vi "TagDashboard.vi"(7 "Name(\"\" to use uuid)":string="UI.Dashboard") -> ()   [LabVIEW 2020, in "CSM-TagDashboard.lvlib"]
doc: "------------- lvcsm -------------\n[CSMStates]\nItem 0 = \"Idle\"\nItem 1 = \"CSM Documentation\"\nItem 2 = \"VI Reference\"\nItem 3 = \"Error Handler\"\nItem 4 = \"Critical Error\"\nItem 5 = \"Target Timeout Error\"\nItem 6 = \"Target Error\"\nItem 7 = \"Async Response\"\nItem 8 = \"Response\"\nItem 9 = \"Async Message Posted\"\nItem 10 = \"Initialize Core Data\"\nItem 11 = \"Exit\"\nItem 12 = \"Data: Initialize\"\nItem 13 = \"Data: Update Indicators\"\nItem 14 = \"Data: Load Attributes\"\nItem 15 = \"Data: Save Attributes\"\nItem 16 = \"Data: Cleanup\"\nItem 17 = \"Macro: Initialize\"\nItem 18 = \"Macro: Exit\"\nItem 19 = \"API: Start Refreshing\"\nItem 20 = \"API: Stop Refreshing\"\nItem 21 = \"Action: Insert TestStandOI\"\nItem 22 = \"Action: Relocate Boolean Switchs\"\nItem 23 = \"Action: 修改bool状态\"\nItem 24 = \"Action: Sync Bool Value with DB\"\nItem 25 = \"Action: 更新当前测试名称\"\nItem 26 = \"Action: Refresh Waveform\"\nItem 27 = \"Action: Refresh Check\"\nItem 28 = \"Action: Resize Array\"\n\n[CSMStatus]\nItem 0 = \"Error Occurred@Error Handler\"\nItem 1 = \"电磁阀状态修改@Action: 修改bool状态\""
uses:
  CSM-TagDashboard.lvlib
  a029ab59-1b26-456a-9f2f-fd23f89c2af1.vi
  67aca029-dc61-4838-a765-978c85277e00.vi
  07294343-d0f4-4418-a8a6-c52ea02f7694.vi
  <userlib>/_NEVSTOP/TagDB/_Support/DataAccess/TagDB Ref to DVR.vi
  <userlib>/_NEVSTOP/Communicable State Machine(CSM)/AdvanceAPI/CSM - Revert Arguments-Safe String.vi
  <userlib>/_NEVSTOP/Communicable State Machine(CSM)/_Shared/Trim Single-line Text.vi
  <userlib>/_NEVSTOP/Communicable State Machine(CSM)/AdvanceAPI/CSM - Make String Arguments Safe.vi
  <userlib>/_NEVSTOP/Communicable State Machine(CSM)/AdvanceAPI/CSM - Break Down Multiple States String.vi
  <userlib>/_NEVSTOP/Communicable State Machine(CSM)/AdvanceAPI/CSM - Compact Multiple States.vi
  <userlib>/_NEVSTOP/Communicable State Machine(CSM)/AdvanceAPI/CSM - Keywords.vi
  <userlib>/_NEVSTOP/Communicable State Machine(CSM)/addons/API-String-Arugments-Support/_Support/Convert API String Arguments to Data(variant).vi
  <userlib>/_NEVSTOP/Communicable State Machine(CSM)/AdvanceAPI/CSM - List Modules.vi
  <userlib>/_NEVSTOP/Communicable State Machine(CSM)/Communicable State Machine.lvlib
  <userlib>/_NEVSTOP/TagDB/TagDB.lvlib
panel:
  out "Tags":string[](array[string])
  out "TagDB":refnum<k1>
  out "Prompt":string="Power by CSM, NEVSTOP-LAB\nUnlicensed Version - 0.0min Trial Left"
  out "Dashboard":T1(array[cluster])
  in  "Num Rows":i16=10
  in  "Num Col":i16=8
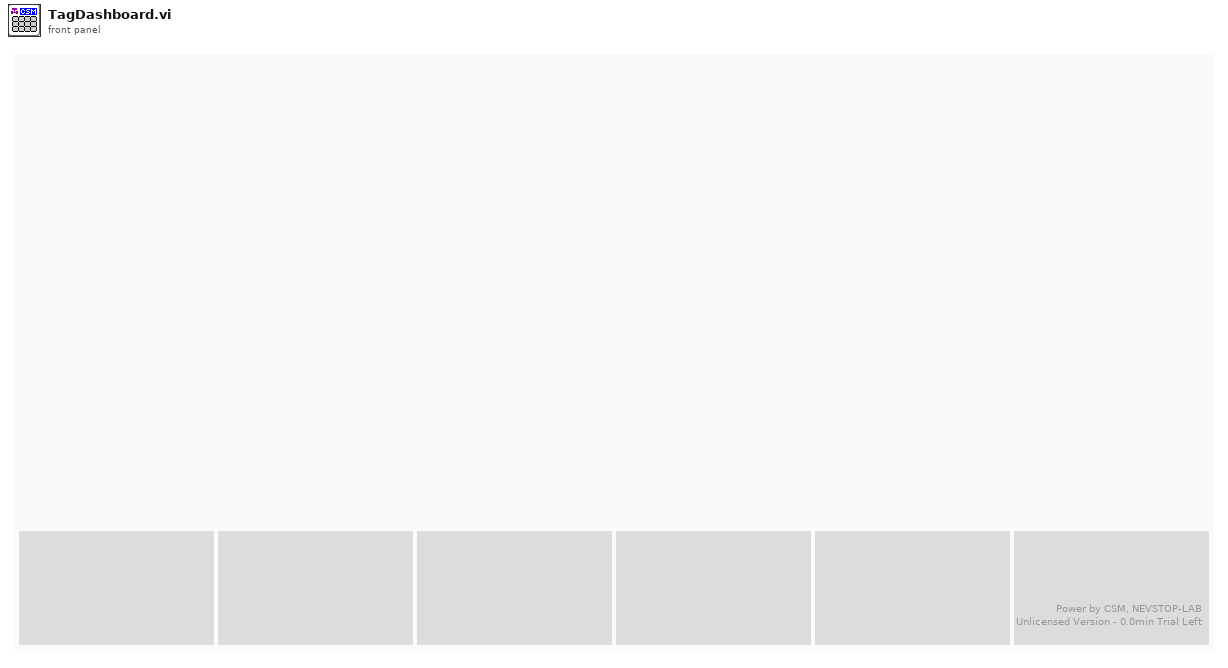
[diagram p1: front panel]
types:
  T1 = cluster{"Label":string, "Value":string, "String":string}[][]
  T2 = cluster{"Label Font Size":i32, "Data Font Size":i32, "String Font Size":i32}
  T3 = cluster{"DataName(dup)":string, "Output String":string, "Unit":string}[][]
  T4 = typedef "LVPositionTypeDef.ctl" = cluster{"Left":i32, "Top":i32}
  T5 = typedef "LVBoundsTypeDef.ctl" = cluster{"Width":u32, "Height":u32}
  T6 = cluster{"Position":T4, "Bounds":T5, "Num Col":i16, "Num Rows":i16, "Cluster":cluster{"Label Font Size":i32, "Data Font Size":i32, "String Font Size":i32}, "Width":u32, "Height":u32}
  T7 = enum32{"Invalid", "Standard", "Closed", "Hidden", "Minimized", "Maximized"}
  T8 = enum32{"invalid app kind", "Development System", "Run Time System", "Student Edition", "Embedded LabVIEW", "Evaluation", "Custom"}
  T9 = typedef "Communicable State Machine.lvlib/_CSM_Response Source Message.ctl" = cluster{"‘State":string, "’Arguments":string, "’Error":errorcluster}
  T10 = cluster{"Current VI Reference":refnum<vi>, "Close Panel on Exit?":bool}
  T11 = cluster{"Core":cluster{"Current VI Reference":refnum<vi>, "Close Panel on Exit?":bool}, "Tags":string[], "Size":cluster{"Cols":i16, "Rows":i16}}
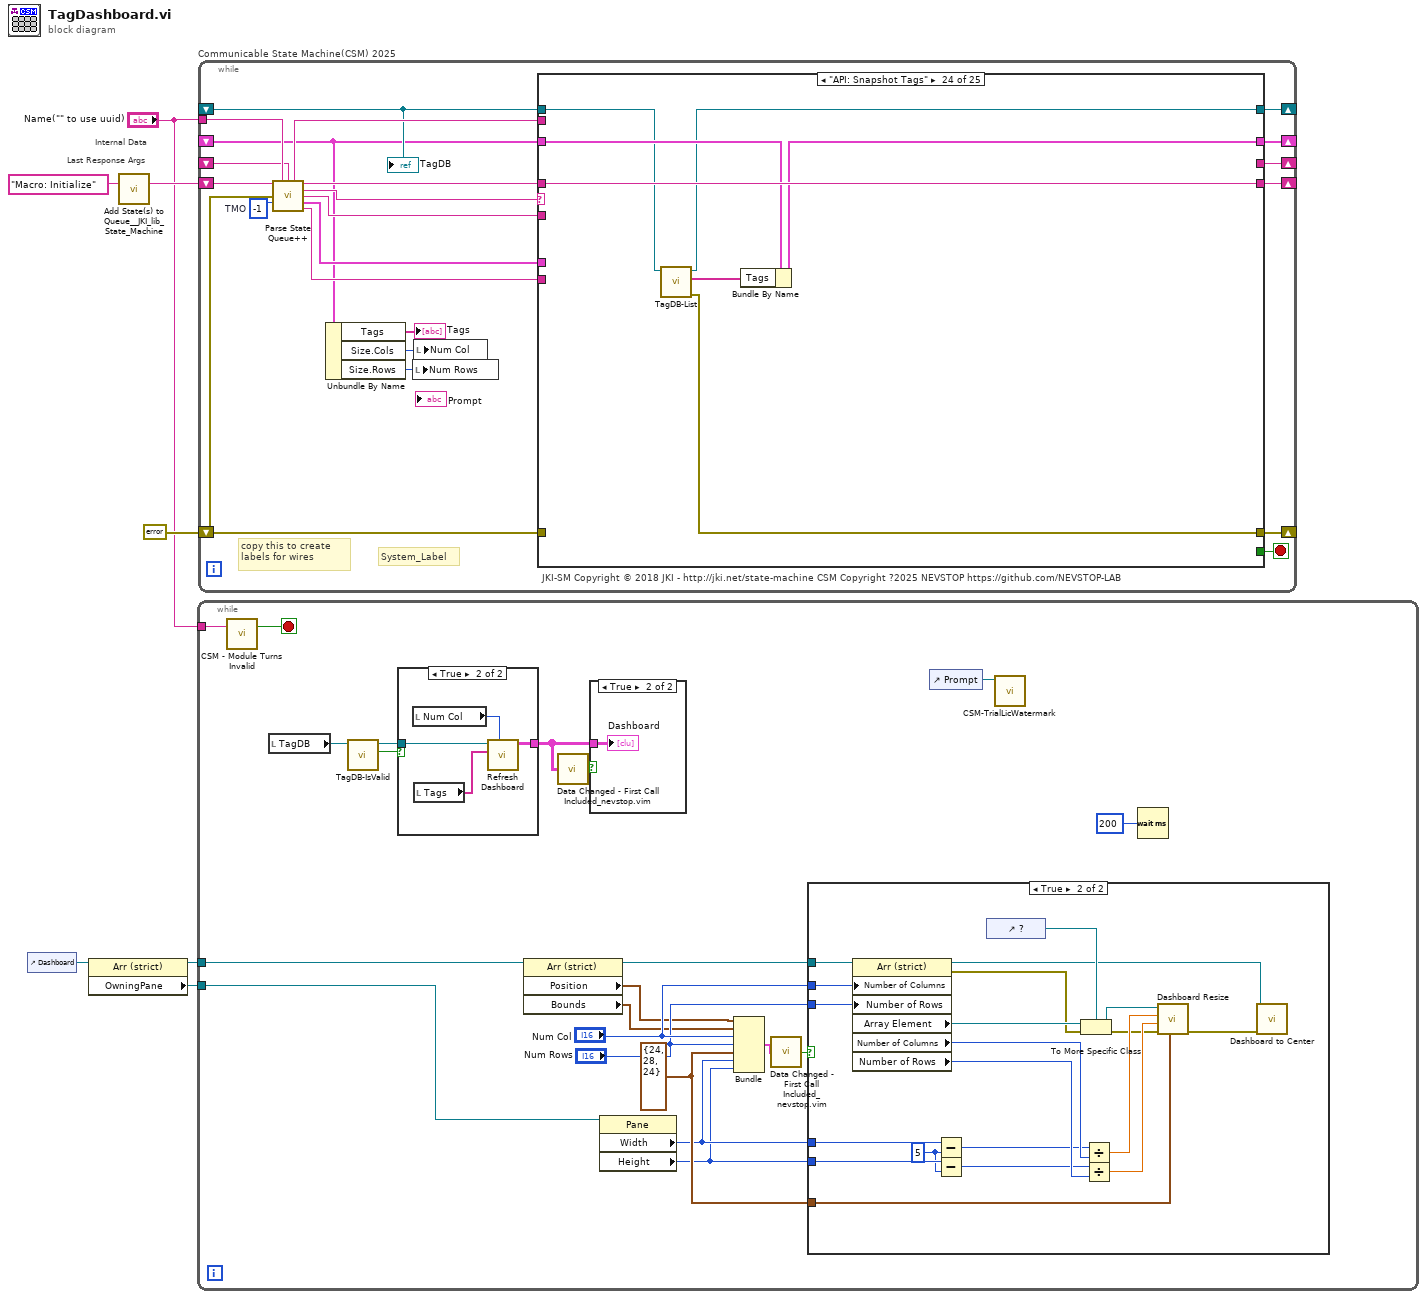
[diagram p0: block diagram]
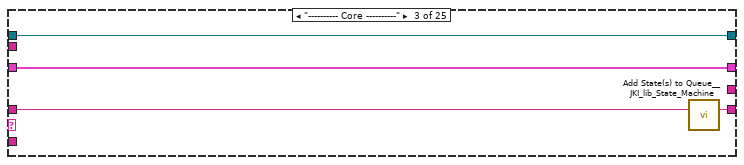
[diagram p7: hidden frame]
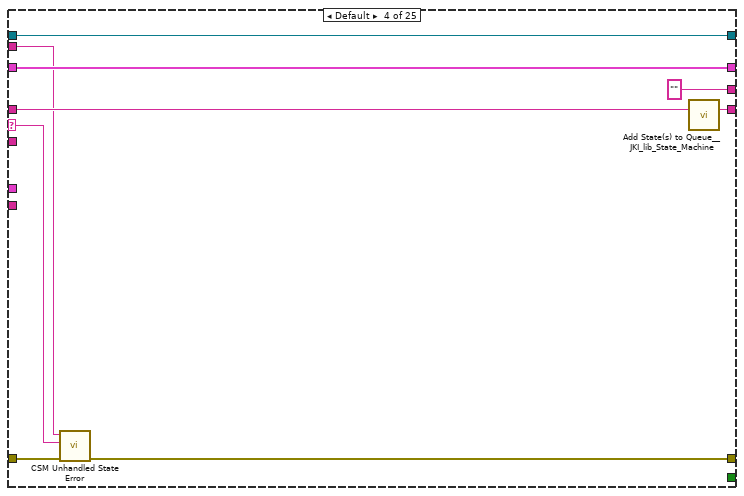
[diagram p8: hidden frame]
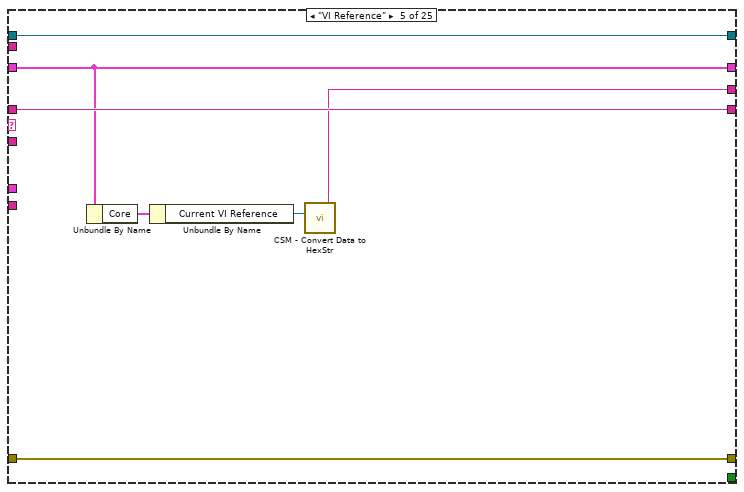
[diagram p9: hidden frame]
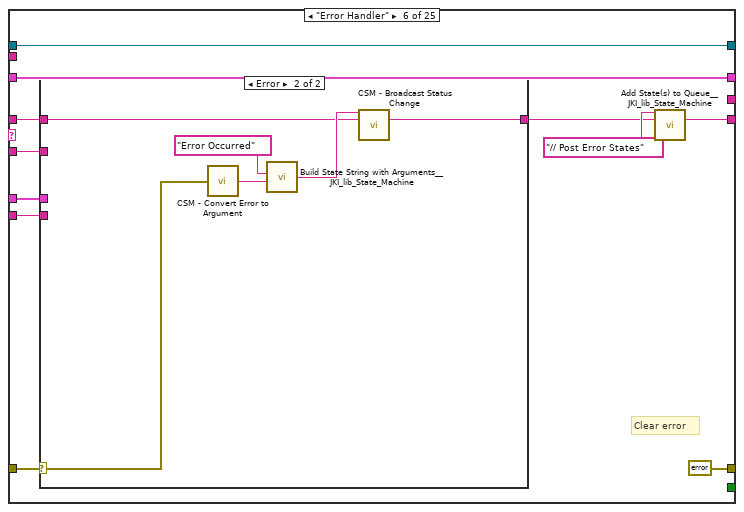
[diagram p10: hidden frame]
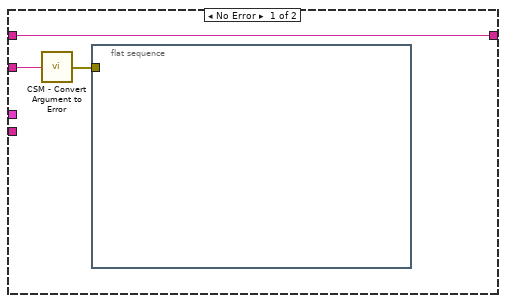
[diagram p11: hidden frame]
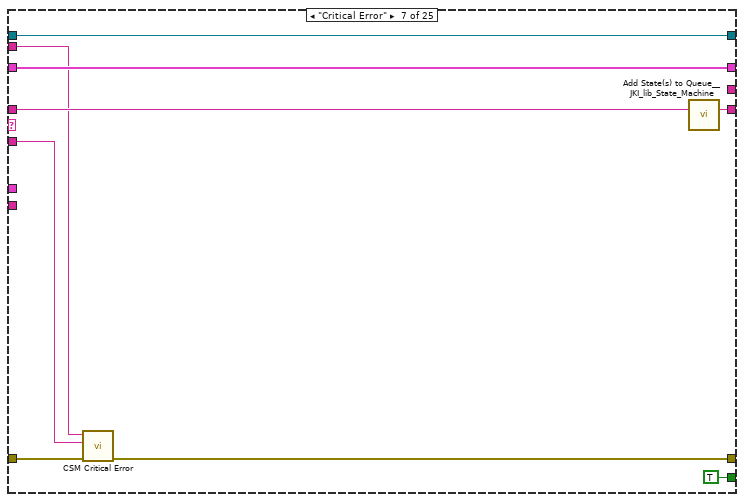
[diagram p12: hidden frame]
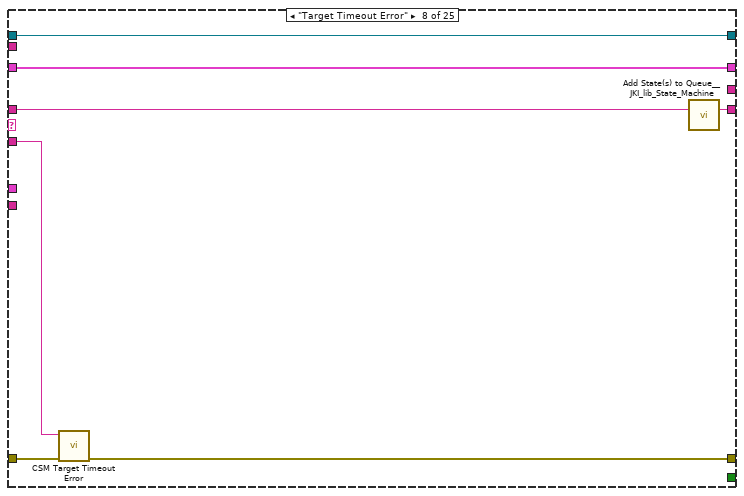
[diagram p13: hidden frame]
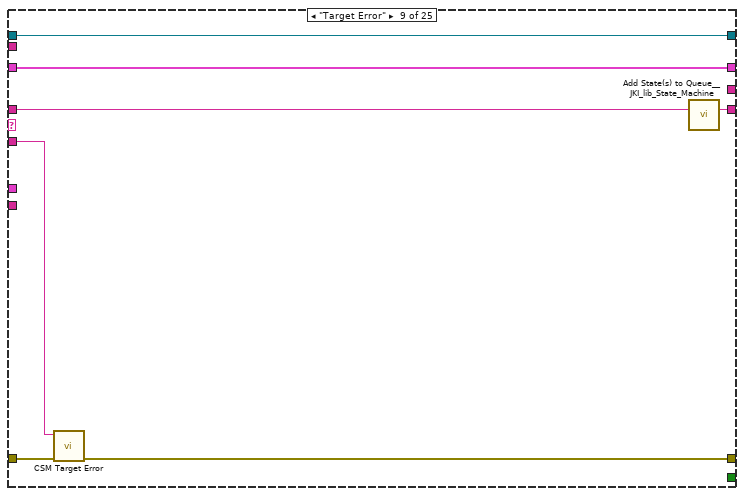
[diagram p14: hidden frame]
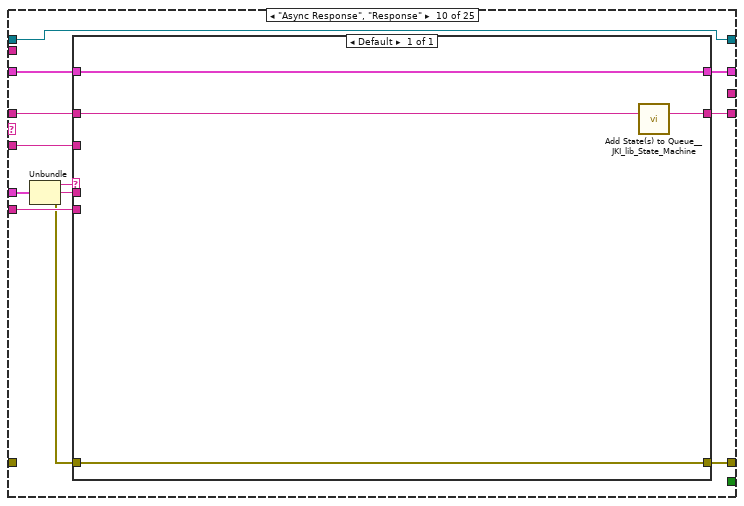
[diagram p15: hidden frame]
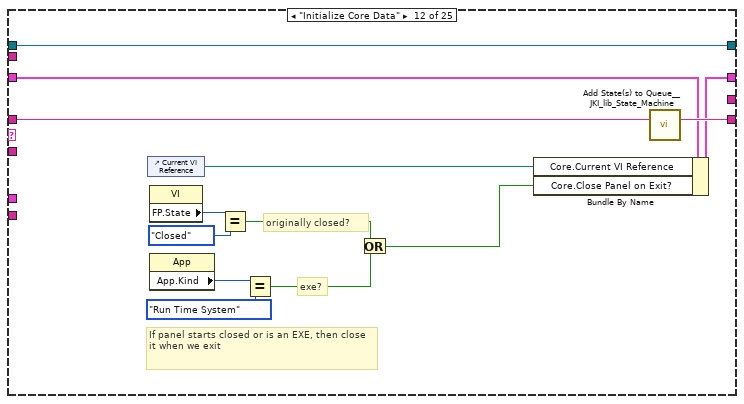
[diagram p17: hidden frame]
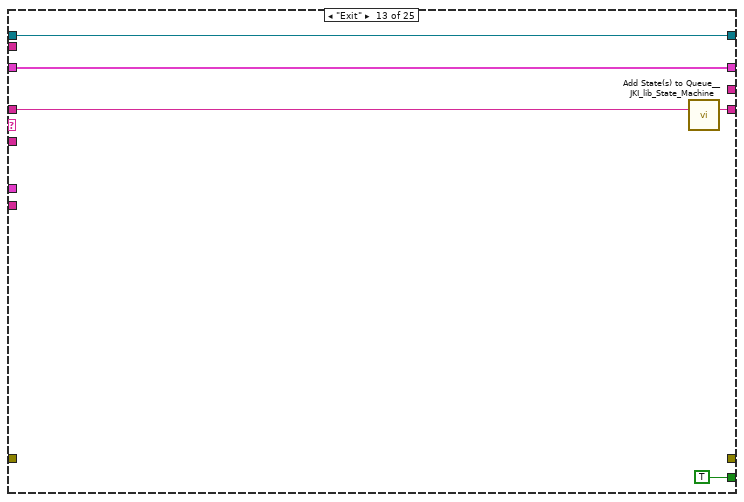
[diagram p18: hidden frame]
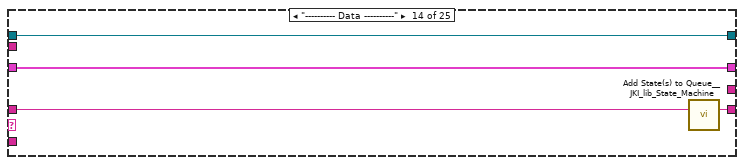
[diagram p19: hidden frame]
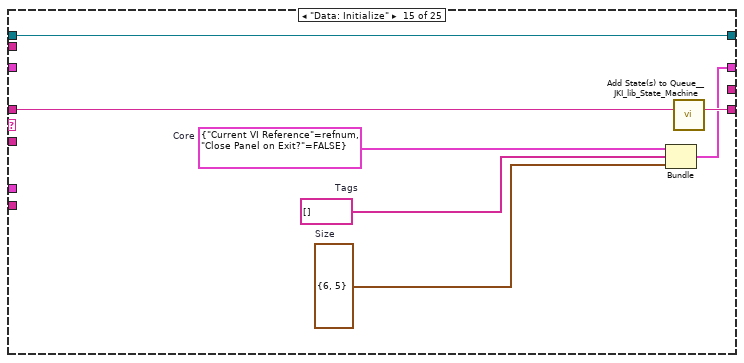
[diagram p20: hidden frame]
diagram:
  # "Last Response Args"
  # "Internal Data"
  n1 = control-ref of="Dashboard"() -> (w4:refnum<vi>)
  n2 = property class="Arr (strict)"(reference=w4) -> (reference out=w3:refnum<vi>, "OwningPane"=w2:refnum<vi>)  [unwired: 1 in, 1 out]
  n3 = call <vilib>:"Add State(s) to Queue__JKI_lib_State_Machine.vi"("State(s) in (\"\")"="Macro: Initialize" ("Init State(\"Macro: Initialize\")")) -> ("States Out"=w7:string)  [unwired: 14 in]
  n4 = while {
    tunnel: "Name(\"\" to use uuid)" -> [w28]
    tunnel: w3 -> [w14]
    tunnel: w2 -> [w13]
    stop <- w27 stop-if-true
    w20 = T2 {"Label Font Size"=24, "Data Font Size"=28, "String Font Size"=24} ("Cluster")
    n5 = call <userlib>:"CSM - Module Turns Invalid.vi"("CSM Name"=w28) -> ("Turn Invalid (Exit)?"=w27:bool)  [unwired: 2 in]
    n6 = local read "TagDB"() -> (w25:refnum<k1>)
    n7 = call <userlib>:"TagDB-IsValid.vi"("TagDB"=w25) -> ("valid TagDB?"=w23:bool, "TagDB(dup)"=w24:refnum<k1>)  [unwired: 8 in, 1 out]
    n8 = case shown="True" w23 {
      tunnel: [_ w33] -> w19
      tunnel: w24 -> [_ w31]
      frame False {
      }
      frame True {
        n9 = local read "Num Col"() -> (w32:i16)
        n10 = local read "Tags"() -> (w30:string[])
        n11 = call "Refresh Dashboard.vi"("Num Col"=w32, "appended array"=w30, "Refnum in"=w31) -> ("Array"=w33:T3)  [unwired: 8 in]
      }
    }
    n12 = property class="Arr (strict)"(reference=w14) -> (reference out=w11:refnum<vi>, "Position"=w9:T4, "Bounds"=w10:T5)  [unwired: 1 in, 1 out]
    n13 = call "Data Changed - First Call Included_nevstop.vim"("Variant"=w19) -> ("Changed"=w18:bool)
    n14 = case shown="True" w18 {
      tunnel: w19 -> [_ w29]
      frame False {
      }
      frame True {
        "Dashboard" <- w29
      }
    }
    n15 = property on="Property Node" class="Pane"(reference=w13) -> ("Width"=w17:u32, "Height"=w16:u32)  [unwired: 1 in, 2 out]
    n16 = Bundle("Position"=w9, "Bounds"=w10, "Num Col"="Num Col", "Num Rows"="Num Rows", "Cluster"=w20, "Width"=w17, "Height"=w16) -> (w15:T6)  [unwired: 1 in]
    n17 = call "Data Changed - First Call Included_nevstop.vim"("Variant"=w15) -> ("Changed"=w8:bool)
    n18 = case shown="True" w8 {
      tunnel: "Num Col" -> [_ w42]
      tunnel: "Num Rows" -> [_ w41]
      tunnel: w20 -> [_ w40]
      tunnel: w11 -> [_ w39]
      tunnel: w17 -> [_ w38]
      tunnel: w16 -> [_ w37]
      frame False {
      }
      frame True {
        w34 = u32 5 ("y")
        n19 = property on="Property Node" class="Arr (strict)"(reference=w39, "Number of Columns"=w42, "Number of Rows"=w41) -> (reference out=w43:refnum<vi>, error out=w51:errorcluster, "Array Element"=w53:refnum<vi>, "Number of Columns"=w52:u32, "Number of Rows"=w50:u32)  [unwired: 1 in]
        n20 = Subtract(x=w38, y=w34) -> (x-y=w36:u32)
        n21 = Subtract(x=w37, y=w34) -> (x-y=w35:u32)
        n22 = control-ref of="?"() -> (w45:refnum<vi>)
        n23 = To More Specific Class(target class=w45, reference=w53, error in=w51) -> (specific class reference=w49:refnum<vi>, error out=w46:errorcluster)
        n24 = Divide(x=w36, y=w52) -> (x/y=w48:dbl)
        n25 = Divide(x=w35, y=w50) -> (x/y=w47:dbl)
        n26 = call "Dashboard Resize.vi"("Cluster"=w40, "error in (no error)"=w46, "Cluster Size:Height"=w47, "Cluster Size:Width"=w48, "ClusterRef"=w49) -> ("error out"=w44:errorcluster)  [unwired: 4 in, 2 out]
        n27 = call "Dashboard to Center.vi"("error in (no error)"=w44, "Control Ref"=w43) -> ()  [unwired: 9 in, 1 out]
      }
    }
    n28 = control-ref of="Prompt"() -> (w12:refnum<vi>)
    n29 = call <userlib>:"CSM-TrialLicWatermark.vi"("TrialLicWatermark"=w12) -> ()  [unwired: 8 in, 3 out]
    n30 = Wait (ms)(milliseconds to wait=u32 200) -> ()  [unwired: 1 out]
  }
  n31 = while "Communicable State Machine(CSM) 2025" {
    shift-right: [w70] -> _
    shift-left: _ -> [w57]
    shift-right: [w73] -> _
    shift-left: errorcluster {"status"=FALSE, "code"=0, "source"=""} ("error out") -> [w60]
    shift-right: [w72] -> _
    shift-left: w7 -> [w74]
    tunnel: "Name(\"\" to use uuid)" -> [w67]
    shift-right: [w68] -> _
    shift-left: _ -> [w62]
    shift-right: [w59] -> _
    shift-left: _ -> [w58]
    stop <- w71 stop-if-true
    w69 = -1  # TMO
    # "JKI-SM Copyright © 2018 JKI - http://jki.net/state-machine CSM Copyright ?2025 NEVSTOP https://github.com/NEVSTOP-LAB"
    # "copy this to create labels for wires"
    # "System_Label"
    n32 = call <userlib>:"Parse State Queue++.vi"("State Queue"=w74, "Name (\"\" to Use UUID)"=w67, "Response Arguments"=w62, "Previous Error"=w60, "Dequeue (1 ms)"=w69) -> ("Name Used"=w61:string, "Remaining States"=w75:string, "Current State"=w63:string, "Arguments"=w64:string, "Additional Information"=w65:T9, "Source CSM"=w66:string)  [unwired: 5 in]
    n33 = Unbundle By Name(w57) -> ("Tags"=→"Tags":string[], "Size.Cols"=w55:i16, "Size.Rows"=w54:i16)
    n34 = local write "Num Rows"(w54) -> ()
    n35 = local write "Num Col"(w55) -> ()
    n36 = case shown="\"API: Snapshot Tags\"" w63 {
      selector: w63 -> [_ _ _ w90 _ _ _ _ _ _ _ _ _ _ _ _ _ _ _ _ _ _ _ _ _]
      tunnel: w75 -> [w77 w81 w85 w94 w100 w106 w130 w137 w144 w155 w163 w176 w181 w185 w192 w195 w202 w206 w211 w218 w221 w226 w233 w241 w245]
      tunnel: w64 -> [_ _ _ _ _ w105 w126 w134 w141 w149 _ _ _ _ _ _ _ _ _ _ _ w223 w230 _ _]
      tunnel: w57 -> [w78 w80 w83 w92 w99 w111 w128 w135 w142 w153 w162 w170 w179 w183 _ w194 w197 w204 w209 w216 w220 w225 w232 w240 w243]
      tunnel: [_ _ _ w87 w101 errorcluster {"status"=FALSE, "code"=0, "source"=""} ("error out") w123 w132 w139 w156 _ _ _ _ _ _ w198 _ _ _ _ w224 w234 w235 _] -> w73
      tunnel: w60 -> [_ _ _ w88 w101 w109 w124 w133 w140 _ _ _ _ _ _ _ w199 _ _ _ _ _ w234 _ _]
      tunnel: [w77 w81 w84 w93 w100 w107 w129 w136 w143 w154 w163 w175 w180 w184 w191 w195 w201 w205 w210 w217 w221 w226 w233 w241 w244] -> w72
      tunnel: [_ _ _ _ _ _ TRUE _ _ _ _ _ TRUE _ _ _ _ _ _ _ _ _ _ _ _] -> w71
      tunnel: [w78 w80 w83 w92 w99 w111 w128 w135 w142 w152 w162 w174 w179 w183 w190 w194 w197 w204 w209 w216 w220 w225 w228 w237 w243] -> w70
      tunnel: w66 -> [_ _ _ _ _ w104 _ _ _ w150 _ _ _ _ _ _ _ _ _ _ _ _ _ _ _]
      tunnel: w65 -> [_ _ _ _ _ w103 _ _ _ w151 _ _ _ _ _ _ _ _ _ _ _ _ _ _ _]
      tunnel: [_ _ _ "" w96 _ _ _ _ _ _ _ _ _ _ _ _ _ _ _ _ _ _ _ _] -> w68
      tunnel: w61 -> [_ _ _ w89 _ _ w125 _ _ _ _ _ _ _ _ _ _ _ _ _ _ _ _ _ _]
      tunnel: [w76 w79 w82 w86 w95 w102 w122 w131 w138 w145 w161 w164 w177 w182 w187 w193 w196 w203 w207 w212 w219 w222 w231 w238 w242] -> w59
      tunnel: w58 -> [w76 w79 w82 w86 w95 w102 w122 w131 w138 w145 w161 w164 w177 w182 w187 w193 w196 w203 w207 w212 w219 _ w231 w239 w242]
      frame "", "Idle" {
      }
      frame "CSM Documentation" {
      }
      frame "---------- Core ----------" {
        n37 = call <vilib>:"Add State(s) to Queue__JKI_lib_State_Machine.vi"("State(s) in (\"\")"=w85) -> ("States Out"=w84:string)  [unwired: 14 in]
      }
      frame Default {
        n38 = call <userlib>:"CSM Unhandled State Error.vi"("error in (no error)"=w88, "Undefined State"=w90, "CSM Name"=w89) -> ("error out"=w87:errorcluster)  [unwired: 8 in]
        n39 = call <vilib>:"Add State(s) to Queue__JKI_lib_State_Machine.vi"("State(s) in (\"\")"=w94) -> ("States Out"=w93:string)  [unwired: 14 in]
      }
      frame "VI Reference" {
        n40 = Unbundle By Name(w99) -> ("Core"=w98:T10)
        n41 = Unbundle By Name(w98) -> ("Current VI Reference"=w97:refnum<vi>)
        n42 = call <userlib>:"CSM - Convert Data to HexStr.vi"("Variant"=w97) -> ("HEX String (0-9,A-F)"=w96:string)  [unwired: 8 in]
      }
      frame "Error Handler" {
        # "Clear error"
        n43 = case shown="Error" w109 {
          selector: w109 -> [_ w116]
          tunnel: [w115 w118] -> w108
          tunnel: w106 -> [w115 w117]
          tunnel: w105 -> [w114 _]
          tunnel: w104 -> [_ _]
          tunnel: w103 -> [_ _]
          frame No Error {
            n44 = call <userlib>:"CSM - Convert Argument to Error.vi"("Argument"=w114) -> ("Error"=w113:errorcluster)  [unwired: 4 in]
            n45 = flat-sequence {
              tunnel: w113 -> [_]
              frame #0 {
              }
            }
          }
          frame Error {
            n46 = call <userlib>:"CSM - Convert Error to Argument.vi"("Error"=w116) -> ("Argument"=w120:string)  [unwired: 4 in]
            n47 = call <vilib>:"Build State String with Arguments__JKI_lib_State_Machine.vi"("Arguments (\"\")"=w120, "State"="Error Occurred" ("Status with Arguments")) -> ("State with Arguments"=w119:string)  [unwired: 4 in]
            n48 = call <userlib>:"CSM - Broadcast Status Change.vi"("Status With Arguments"=w119, "State Queue"=w117) -> ("Remaining States"=w118:string)  [unwired: 13 in]
          }
        }
        n49 = call <vilib>:"Add State(s) to Queue__JKI_lib_State_Machine.vi"("State(s) in Front (\"\")"="// Post Error States", "State(s) in (\"\")"=w108) -> ("States Out"=w107:string)  [unwired: 13 in]
      }
      frame "Critical Error" {
        n50 = call <userlib>:"CSM Critical Error.vi"("error in (no error)"=w124, "Arugments (As Reason)"=w126, "CSM Name"=w125) -> ("error out"=w123:errorcluster)  [unwired: 8 in]
        n51 = call <vilib>:"Add State(s) to Queue__JKI_lib_State_Machine.vi"("State(s) in (\"\")"=w130) -> ("States Out"=w129:string)  [unwired: 14 in]
      }
      frame "Target Timeout Error" {
        n52 = call <userlib>:"CSM Target Timeout Error.vi"("error in (no error)"=w133, "Arguments (As CSM Name)"=w134) -> ("error out"=w132:errorcluster)  [unwired: 9 in]
        n53 = call <vilib>:"Add State(s) to Queue__JKI_lib_State_Machine.vi"("State(s) in (\"\")"=w137) -> ("States Out"=w136:string)  [unwired: 14 in]
      }
      frame "Target Error" {
        n54 = call <userlib>:"CSM Target Error.vi"("error in (no error)"=w140, "Arguments (As CSM Name)"=w141) -> ("error out"=w139:errorcluster)  [unwired: 9 in]
        n55 = call <vilib>:"Add State(s) to Queue__JKI_lib_State_Machine.vi"("State(s) in (\"\")"=w144) -> ("States Out"=w143:string)  [unwired: 14 in]
      }
      frame "Async Response", "Response" {
        n56 = Unbundle(w151) -> ("‘State"=w148:string, "’Arguments"=w147:string, "’Error"=w146:errorcluster)
        n57 = case shown="Default" w148 {
          tunnel: [w157] -> w154
          tunnel: w155 -> [w158]
          tunnel: [w160] -> w152
          tunnel: w153 -> [w160]
          tunnel: [w159] -> w156
          tunnel: w146 -> [w159]
          tunnel: w150 -> [_]
          tunnel: w149 -> [_]
          tunnel: w147 -> [_]
          frame Default {
            n58 = call <vilib>:"Add State(s) to Queue__JKI_lib_State_Machine.vi"("State(s) in (\"\")"=w158) -> ("States Out"=w157:string)  [unwired: 14 in]
          }
        }
      }
      frame "Async Message Posted" {
      }
      frame "Initialize Core Data" {
        # "originally closed?"
        # "exe?"
        # "If panel starts closed or is an EXE, then close it when we exit"
        n59 = control-ref of="Current VI Reference"() -> (w168:refnum<vi>)
        n60 = property class="VI"() -> ("FP.State"=w167:T7)  [unwired: 2 in, 2 out]
        n61 = property class="App"() -> ("App.Kind"=w173:T8)  [unwired: 2 in, 2 out]
        n62 = Equal?(x=w167, y=T7."Closed" ("Front Panel Window:State")) -> (x = y?=w165:bool)
        n63 = Equal?(x=w173, y=T8."Run Time System" ("Application:Kind")) -> (x = y?=w171:bool)
        n64 = Or(x=w165, y=w171) -> (x .or. y?=w169:bool)
        n65 = Bundle By Name(cluster=w170, "Core.Current VI Reference"=w168, "Core.Close Panel on Exit?"=w169) -> (w174:T11)
        n66 = call <vilib>:"Add State(s) to Queue__JKI_lib_State_Machine.vi"("State(s) in (\"\")"=w176) -> ("States Out"=w175:string)  [unwired: 14 in]
      }
      frame "Exit" {
        n67 = call <vilib>:"Add State(s) to Queue__JKI_lib_State_Machine.vi"("State(s) in (\"\")"=w181) -> ("States Out"=w180:string)  [unwired: 14 in]
      }
      frame "---------- Data ----------" {
        n68 = call <vilib>:"Add State(s) to Queue__JKI_lib_State_Machine.vi"("State(s) in (\"\")"=w185) -> ("States Out"=w184:string)  [unwired: 14 in]
      }
      frame "Data: Initialize" {
        w186 = cluster{"Cols":i16, "Rows":i16} {"Cols"=6, "Rows"=5}  # Size
        w188 = string[] []  # Tags
        w189 = T10 {"Current VI Reference"=refnum, "Close Panel on Exit?"=FALSE}  # Core
        n69 = Bundle("Core"=w189, "Tags"=w188, "Size"=w186) -> (w190:T11)  [unwired: 1 in]
        n70 = call <vilib>:"Add State(s) to Queue__JKI_lib_State_Machine.vi"("State(s) in (\"\")"=w192) -> ("States Out"=w191:string)  [unwired: 14 in]
      }
      frame "Data: Update Indicators" {
      }
      frame "Data: Cleanup" {
        n71 = Unbundle By Name(w197) -> ("Core.Current VI Reference"=w200:refnum<vi>)
        n72 = Close Reference(reference=w200, error in (no error)=w199) -> (error out=w198:errorcluster)
        n73 = call <vilib>:"Add State(s) to Queue__JKI_lib_State_Machine.vi"("State(s) in (\"\")"=w202) -> ("States Out"=w201:string)  [unwired: 14 in]
      }
      frame "---------- Macro ----------" {
        n74 = call <vilib>:"Add State(s) to Queue__JKI_lib_State_Machine.vi"("State(s) in (\"\")"=w206) -> ("States Out"=w205:string)  [unwired: 14 in]
      }
      frame "Macro: Initialize" {
        n75 = call <vilib>:"Add State(s) to Queue__JKI_lib_State_Machine.vi"("State(s) in Front (\"\")"="Data: Initialize\nInitialize Core Data\nData: Update Indicators", "State(s) in (\"\")"=w211) -> ("States Out"=w210:string)  [unwired: 13 in]
      }
      frame "Macro: Exit" {
        n76 = call <vilib>:"Add State(s) to Queue__JKI_lib_State_Machine.vi"("State(s) in Front (\"\")"="//Exit Sub-Modules ", "State(s) at Back (\"\")"="Data: Cleanup\nExit") -> ("States Out"=w214:string)  [unwired: 13 in]
        n77 = call <vilib>:"Add State(s) to Queue__JKI_lib_State_Machine.vi"("State(s) in Front (\"\")"=w214, "State(s) in (\"\")"=w218) -> ("States Out"=w217:string)  [unwired: 13 in]
      }
      frame "---------- API ----------" {
      }
      frame "API: Set TagDB" {
        n78 = call <userlib>:"TagDB-Obtain.vi"("name (unnamed)"=w223) -> ("error out"=w224:errorcluster, "TagDB"=w222:refnum<k1>)  [unwired: 4 in, 1 out]
      }
      frame "API: Set Tags" {
        n79 = call "Convert API String Arguments to Data.vim"("Reference Type"=string[] [] ("Arguments"), "API String"=w230) -> ("Data"=w227:string[])  [unwired: 6 in, 1 out]
        n80 = Bundle By Name(cluster=w232, "Tags"=w227) -> (w228:T11)
      }
      frame "API: Snapshot Tags" {
        n81 = call <userlib>:"TagDB-List.vi"("TagDB"=w239) -> ("error out"=w235:errorcluster, "names"=w236:string[], "TagDB(dup)"=w238:refnum<k1>)  [unwired: 7 in, 1 out]
        n82 = Bundle By Name(cluster=w240, "Tags"=w236) -> (w237:T11)
      }
      frame "---------- Action ----------" {
        n83 = call <vilib>:"Add State(s) to Queue__JKI_lib_State_Machine.vi"("State(s) in (\"\")"=w245) -> ("States Out"=w244:string)  [unwired: 14 in]
      }
    }
    "TagDB" <- w58
  }
